vi "Close Device Reference.vi"(8 "error in (no error)":errorcluster, 10 "Device":refnum<k24>, 11 "KCubeInertialMotorControl in":refnum<k24>) -> (0 "error out":errorcluster)   [LabVIEW 2017]
uses:
  D:/upwork/Laser Measurement Tool/Laser/tests/KIM101/Thorlabs.MotionControl.Controls.dll
  Thorlabs.MotionControl.Controls.dll
  D:/upwork/Laser Measurement Tool/Laser/tests/KIM101/Thorlabs.MotionControl.KCube.InertialMotorCLI.dll
  Thorlabs.MotionControl.KCube.InertialMotorCLI.dll
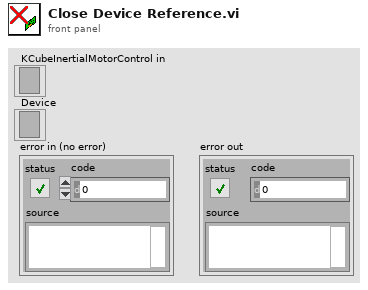
[diagram p1: front panel]
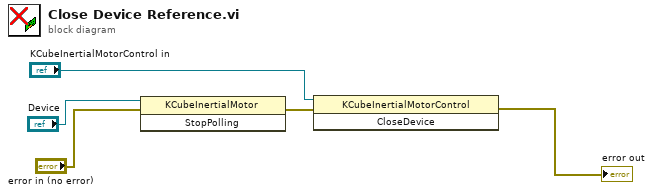
[diagram p0: block diagram]
diagram:
  n1 = invoke class="KCubeInertialMotor" method="StopPolling"(reference="Device", error in="error in (no error)") -> (error out=w3:errorcluster)  [unwired: 1 in, 2 out]
  n2 = invoke class="KCubeInertialMotorControl" method="CloseDevice"(reference="KCubeInertialMotorControl in", error in=w3) -> (error out=→"error out":errorcluster)  [unwired: 1 in, 2 out]
